vi "Edit Substeps Digital Output.vi"(8 "error in":errorcluster, 9 "Station No":i32, 10 "DOWrite":T1, 11 "Sequence Context In":refnum<k7>) -> (0 "error out":errorcluster, 2 "DOWrite Out":T1, 3 "Report Text":string)   [LabVIEW 2023, in "LTT_TeststandSteptypes.lvlib"]
uses:
  LTT_TeststandSteptypes.lvlib
  HardwareAbstractionLayer_LVOOP/Digital Output/DO_class/DO DAQ/Control/DO Write Enable.ctl
  HardwareAbstractionLayer_LVOOP/Database/SQL Public VI/Control/DB Options.ctl
  <vilib>/addons/TestStand/_TSUtility.llb/TestStand - Start Modal Dialog (Sequence Context).vi
  <vilib>/addons/TestStand/_TSUtility.llb/TestStand - End Modal Dialog (Sequence Context).vi
  HardwareAbstractionLayer_LVOOP/Database/Database.lvclass
  HardwareAbstractionLayer_LVOOP/Digital Output/DO_class/DO.lvclass
panel:
  in  "Close":bool
  in  "OK":bool
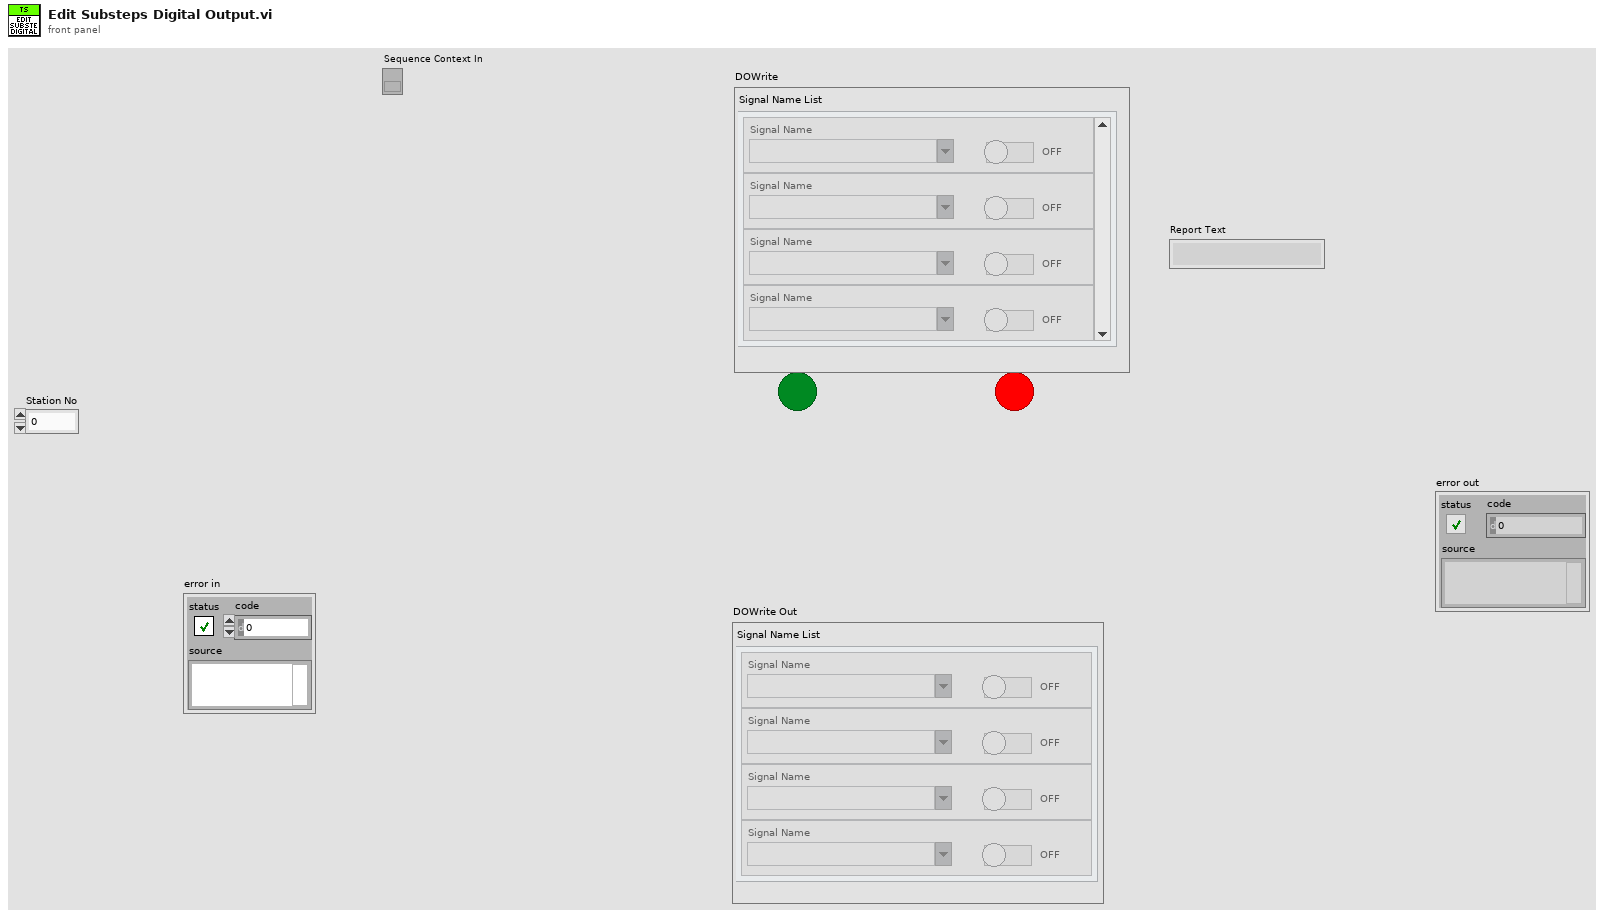
[diagram p1: front panel]
types:
  T1 = typedef "HardwareAbstractionLayer_LVOOP.lvlib/DO.lvclass/DO Write Enable.ctl" = cluster{"Signal Name List":cluster{"Signal Name":string, "Enable Output":bool}[]}
  T2 = typedef "HardwareAbstractionLayer_LVOOP.lvlib/Database.lvclass/DB Options.ctl" = enum16{"Init", "Select Data", "Insert Data", "Update Data", "Delete Data", "Execute Query", "Create Schema", "Create Table", "List Tables", "List Columns", "Close"}
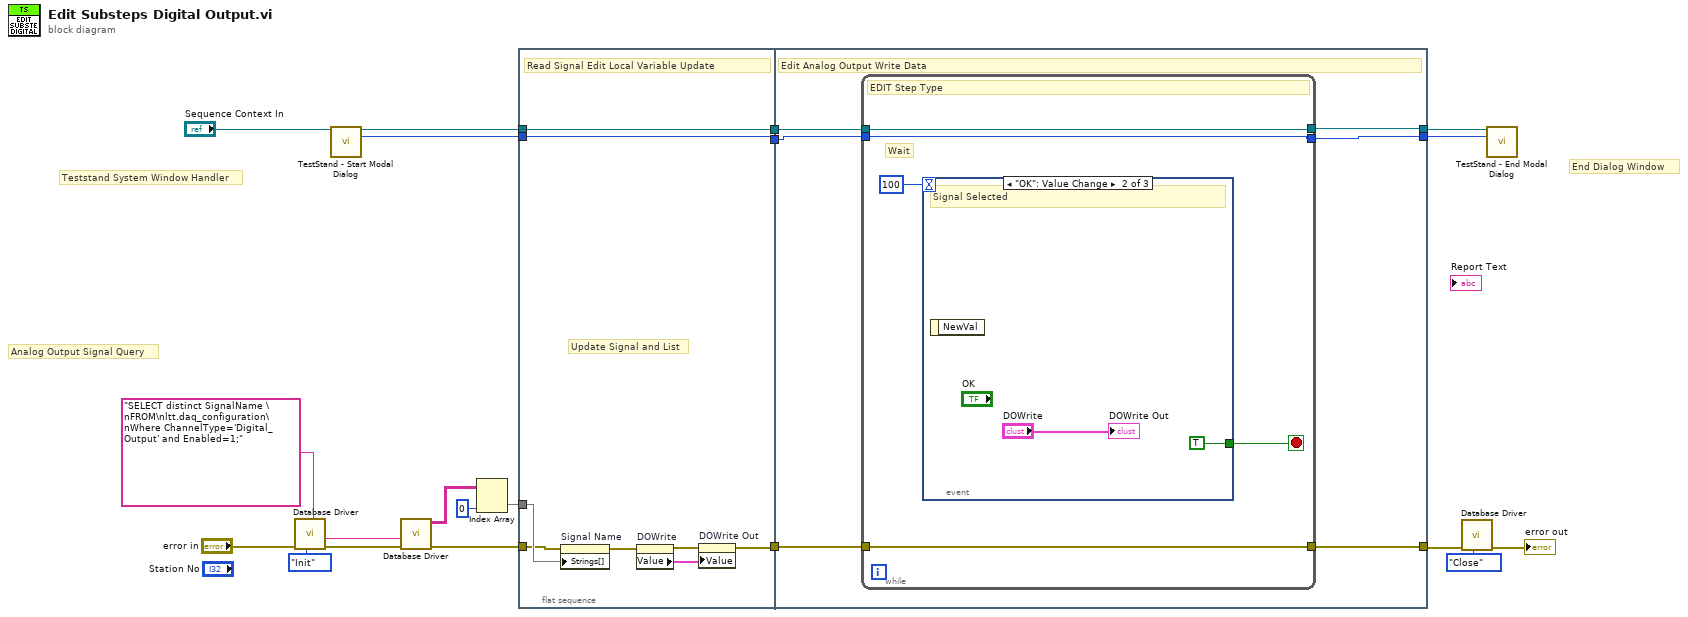
[diagram p0: block diagram]
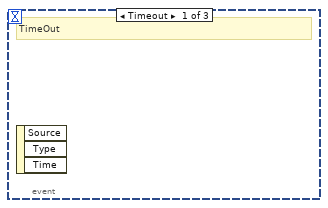
[diagram p2: hidden frame]
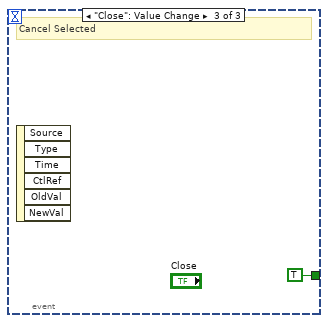
[diagram p3: hidden frame]
diagram:
  # "End Dialog Window"
  # "Teststand System Window Handler"
  # "Analog Output Signal Query"
  n1 = call "Database Driver.vi"("Options"=DB_Options."Init", "error in"="error in") -> ("error out"=w4:errorcluster)  [unwired: 6 in, 3 out]
  n2 = call-poly <vilib>:"TestStand - Start Modal Dialog.vi"("Sequence Context In"="Sequence Context In") -> ("Sequence Context Out"=w14:refnum<k7>, "Modal ID"=w13:i32)  [unwired: 10 in, 3 out]
  n3 = call "Database Driver.vi"("error in"=w4, "SQL query"="SELECT distinct SignalName \nFROM\nltt.daq_configuration\nWhere ChannelType='Digital_Output' and Enabled=1;") -> ("error out"=w10:errorcluster, "data"=w9:string[][])  [unwired: 6 in, 2 out]
  n4 = Index Array(array=w9, index (col)=0 ("disabled index (col)")) -> (element=w8:string[])  [unwired: 1 in]
  n5 = flat-sequence {
    tunnel: w10 -> [w21]
    tunnel: [w20] -> w19
    tunnel: w14 -> [w27]
    tunnel: [w27] -> w17
    tunnel: w8 -> [w25]
    tunnel: w13 -> [w26]
    tunnel: [w26] -> w12
    tunnel: w19 -> [w33]
    tunnel: [w32] -> w18
    tunnel: w17 -> [w31]
    tunnel: [w30] -> w16
    tunnel: w12 -> [w29]
    tunnel: [w28] -> w11
    frame #0 {
      # "Update Signal and List"
      # "Read Signal Edit Local Variable Update"
      n6 = property on="Signal Name" class="CmbBox"(error in=w21, "Strings[]"=w25) -> (error out=w22:errorcluster)  [unwired: 1 in, 1 out]
      n7 = property on="DOWrite" class="Clust (strict)"(error in=w22) -> (error out=w23:errorcluster, "Value"=w24:T1)  [unwired: 1 in, 1 out]
      n8 = property on="DOWrite Out" class="Clust (strict)"(error in=w23, "Value"=w24) -> (error out=w20:errorcluster)  [unwired: 1 in, 1 out]
    }
    frame #1 {
      # "Edit Analog Output Write Data"
      n9 = while {
        tunnel: w33 -> [w38]
        tunnel: [w38] -> w32
        tunnel: w31 -> [w37]
        tunnel: [w37] -> w30
        tunnel: w29 -> [w34]
        tunnel: [w34] -> w28
        stop <- w35 stop-if-true
        # "Wait"
        # "EDIT Step Type"
        n10 = event shown="[1] \"OK\": Value Change" {
          selector: _ -> [_ _ _]
          dyn-events: _ -> [_ _ _]
          timeout: 100 -> [_ _ _]
          tunnel: [_ TRUE ("Stop") TRUE ("Stop")] -> w35
          event Timeout {
            # "TimeOut"
            n11 = event-data() -> ()  [unwired: 1 in, 3 out]
          }
          event "OK": Value Change {
            # "Signal Selected"
            n12 = event-data() -> ()  [unwired: 1 in, 1 out]
            "DOWrite Out" <- "DOWrite"
          }
          event "Close": Value Change {
            # "Cancel Selected"
            n13 = event-data() -> ()  [unwired: 1 in, 6 out]
          }
        }
      }
    }
  }
  n14 = call "Database Driver.vi"("Options"=DB_Options."Close", "error in"=w18) -> ("error out"=→"error out":errorcluster)  [unwired: 6 in, 3 out]
  n15 = call-poly <vilib>:"TestStand - End Modal Dialog.vi"("Sequence Context In"=w16, "Modal ID"=w11) -> ()  [unwired: 13 in, 1 out]
